vi "ExSubToggleReverse.vi"(2 "error in (no error)":errorcluster, 3 "Camera Handle":u32) -> (0 "error out":errorcluster, 1 "Camera Handle":u32)   [LabVIEW 2010]
uses:
  GlobalReverseFlag.vi
  GlobalFlipFlag.vi
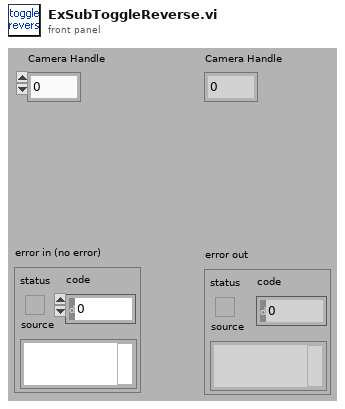
[diagram p1: front panel]
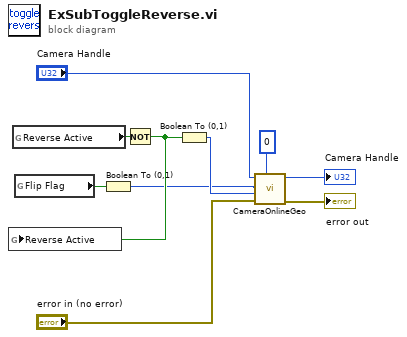
[diagram p0: block diagram]
diagram:
  n1 = global read "GlobalReverseFlag.vi" "Reverse Active"() -> (w10:bool)
  n2 = global read "GlobalFlipFlag.vi" "Flip Flag"() -> (w3:bool)
  n3 = Boolean To (0,1)(Boolean=w3) -> (0, 1=w2:i16)
  n4 = Not(x=w10) -> (.not. x?=w9:bool)
  n5 = global write "GlobalReverseFlag.vi" "Reverse Active"(w9) -> ()
  n6 = Boolean To (0,1)(Boolean=w9) -> (0, 1=w8:i16)
  n7 = call <userlib>:"CameraOnlineGeo.vi"("Camera Handle"="Camera Handle", "Flip Flag"=w2, "Reverse Flag"=w8, "error in"="error in (no error)", "Rotate Flag"=0) -> ("Camera Handle"=→"Camera Handle":u32, "error out"=→"error out":errorcluster)
